vi "Bit Test Pattern.vi"(10 "Bit Pattern(u64)":T1(ring)) -> (1 "lsb-lo(u16)":u16 format="%04x", 2 "msb-lo(u16)":u16 format="%04x", 4 "lsb-hi(u16)":u16 format="%04x", 5 "msb-hi(u16)":u16 format="%04x", 6 "lsb(u32)":u32 format="%08x", 7 "msb(u32)":u32 format="%08x")   [LabVIEW 2025]
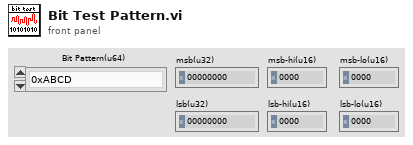
[diagram p1: front panel]
types:
  T1 = enum8{"0xABCD", "0xEEEE", "0xAAAA", "0x5555", "All ONES", "All ZEROES"}
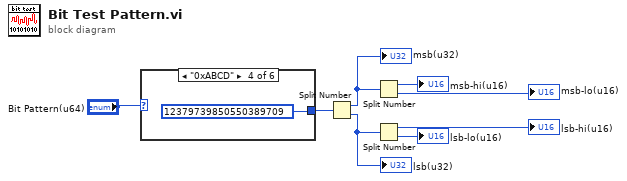
[diagram p0: block diagram]
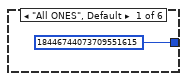
[diagram p2: hidden frame]
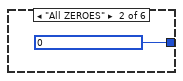
[diagram p3: hidden frame]
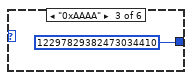
[diagram p4: hidden frame]
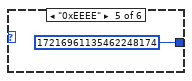
[diagram p5: hidden frame]
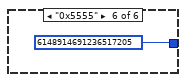
[diagram p6: hidden frame]
diagram:
  n1 = case shown="\"0xABCD\"" "Bit Pattern(u64)" {
    tunnel: [u64 18446744073709551615 u64 0 u64 12297829382473034410 u64 12379739850550389709 u64 17216961135462248174 u64 6148914691236517205] -> w7
    frame "All ONES", Default {
    }
    frame "All ZEROES" {
    }
    frame "0xAAAA" {
    }
    frame "0xABCD" {
    }
    frame "0xEEEE" {
    }
    frame "0x5555" {
    }
  }
  n2 = Split Number(x=w7) -> (hi(x)=w6:u32, lo(x)=w5:u32)
  "msb(u32)" <- w6
  "lsb(u32)" <- w5
  n3 = Split Number(x=w6) -> (hi(x)=→"msb-hi(u16)":u16, lo(x)=→"msb-lo(u16)":u16)
  n4 = Split Number(x=w5) -> (hi(x)=→"lsb-hi(u16)":u16, lo(x)=→"lsb-lo(u16)":u16)
